vi "Write Connected.vi"(8 "error in (no error)":errorcluster, 10 "Connected":refnum<user-event>, 11 "TCPComEvents in":refnum<class "TCPComEvents.lvclass">) -> (0 "error out":errorcluster, 3 "TCPComEvents out":refnum<class "TCPComEvents.lvclass">)   [LabVIEW 2016, in "TCPComEvents.lvclass"]
uses:
  TCPComEvents.lvclass
  TCPComEvents.lvclass/TCPComEvents.ctl
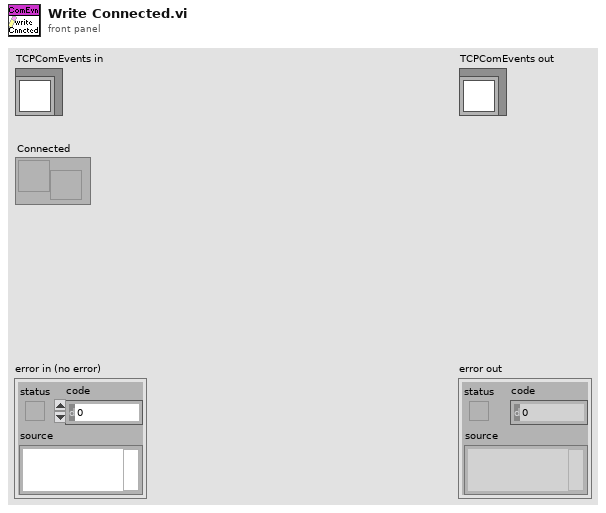
[diagram p1: front panel]
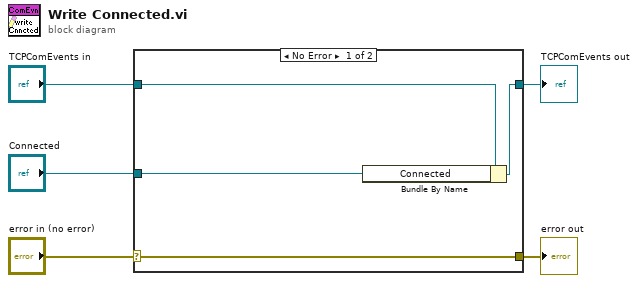
[diagram p0: block diagram]
diagram:
  n1 = case shown="No Error" "error in (no error)" {
    selector: "error in (no error)" -> [w9 w10]
    tunnel: [w9 w10] -> w4
    tunnel: [w7 w11] -> w2
    tunnel: "TCPComEvents in" -> [w8 w11]
    tunnel: "Connected" -> [w6 _]
    frame No Error {
      n2 = Bundle By Name(cluster=w8, "Connected"=w6) -> (w7:refnum<class "TCPComEvents.lvclass">)
    }
    frame Error {
    }
  }
  "error out" <- w4
  "TCPComEvents out" <- w2
